vi "Prepare Input Buffer.vi"(11 "String to Encode":string) -> (3 "Chunked MEssage":u8[][](array[numeric]) format="%02x")   [LabVIEW 2019, in "SHA256.lvlib"]
doc: "Takes a message for SHA-256 hashing and converts it in 512 bit chunks, padding with zeros as necessary and including the length a terminating bit."
uses:
  SHA256.lvlib
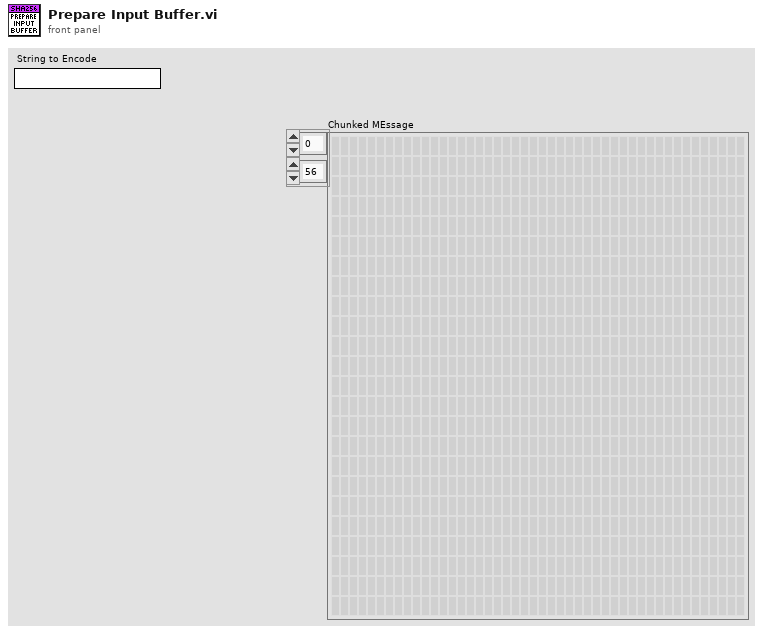
[diagram p1: front panel]
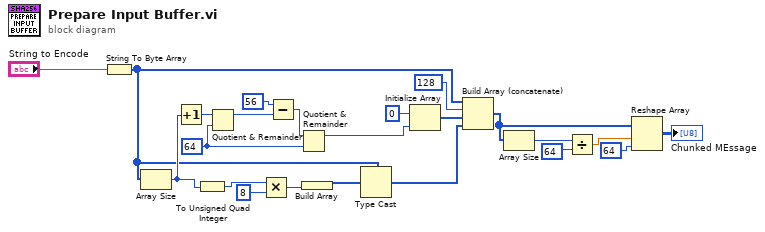
[diagram p0: block diagram]
diagram:
  w9 = 64 ("y")
  n1 = String To Byte Array(string="String to Encode") -> (unsigned byte array=w3:u8[])
  n2 = Array Size(array=w3) -> (size(s)=w8:i32)
  n3 = Increment(x=w8) -> (x+1=w22:i32)
  n4 = To Unsigned Quad Integer(1:w8) -> (0:w7:u64)
  n5 = Quotient & Remainder(x=w22, y=w9) -> (x-y*floor(x/y)=w21:i32)  [unwired: 1 out]
  n6 = Multiply(x=w7, y=u64 8) -> (x*y=w5:u64)
  n7 = Subtract(x=56, y=w21) -> (x-y=w10:i32)
  n8 = Quotient & Remainder(x=w10, y=w9) -> (x-y*floor(x/y)=w1:i32)  [unwired: 1 out]
  n9 = Build Array(w5) -> (w4:u64[])
  n10 = Type Cast(type=w3, x=w4) -> (*(type *) &x=w2:u8[])
  n11 = Initialize Array(u8 0, w1) -> (w18:u8[])
  n12 = Build Array (concatenate)(w3, u8 128, w18, w2) -> (w14:u8[])
  n13 = Array Size(array=w14) -> (size(s)=w16:i32)
  n14 = Divide(x=w16, y=64) -> (x/y=w13:dbl)
  n15 = Reshape Array(w14, w13, 64 ("dimension size")) -> (→"Chunked MEssage":u8[][])
